vi "niScope LabVIEW Error.vi"(2 "instrument handle":u32, 3 "niScope error code (0)":i32 format="%.0x", 5 "error in (no error)":errorcluster) -> (1 "error out":errorcluster)   [LabVIEW 2013]
uses:
  niScope_32.dll
panel:
  out "VI Name":string
  out "instrument handle out":i32
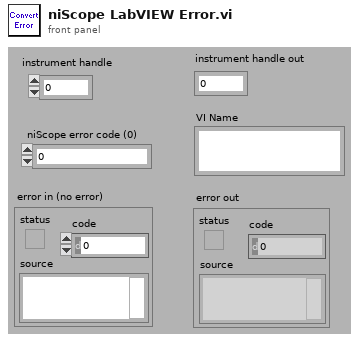
[diagram p1: front panel]
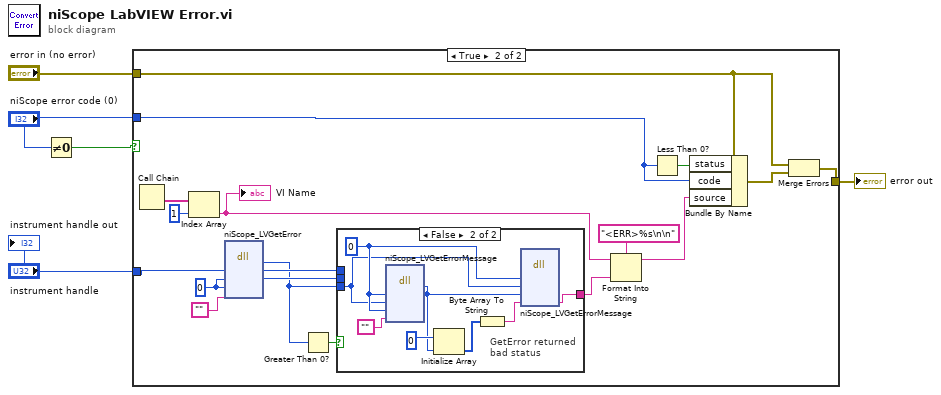
[diagram p0: block diagram]
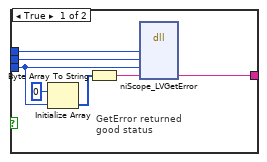
[diagram p3: hidden frame]
diagram:
  n1 = Not Equal To 0?(x="niScope error code (0)") -> (x != 0?=w1:bool)
  n2 = case shown="True" w1 {
    tunnel: "niScope error code (0)" -> [_ w15]
    tunnel: [w6 w11] -> w5
    tunnel: "instrument handle" -> [_ w14]
    tunnel: "error in (no error)" -> [w6 w13]
    frame False {
    }
    frame True {
      w21 = 0
      n3 = Call Chain() -> (call chain=w22:string[])
      n4 = Index Array(array=w22, index=1 ("Index")) -> (element=w7:string)
      "VI Name" <- w7
      n5 = dll-call lib="niScope_*.*" fn="niScope_LVGetError" label="GetError"("instrumentHandle"=w14, "errorCode"=w21, "bufferSize"=w21, "description"="") -> (w8:i32, "instrumentHandle"=w20:u32, "errorCode"=w19:i32)  [unwired: 5 in, 2 out]
      n6 = Greater Than 0?(x=w8) -> (x > 0?=w9:bool)
      n7 = case shown="False" w9 {
        tunnel: w20 -> [w28 _]
        tunnel: w19 -> [w27 _]
        tunnel: [w26 w39] -> w18
        tunnel: w8 -> [w25 w36]
        frame True {
          # "GetError returned\ngood status"
          n8 = Initialize Array(u8 0, w25) -> (w30:u8[])
          n9 = Byte Array To String(unsigned byte array=w30) -> (string=w29:string)
          n10 = dll-call lib="niScope_*.*" fn="niScope_LVGetError" label="GetError"("instrumentHandle"=w28, "errorCode"=w27, "bufferSize"=w25, "description"=w29) -> ("description"=w26:string)  [unwired: 7 in, 2 out]
        }
        frame False {
          w38 = 0 ("instrumentHandle")
          # "GetError returned\nbad status"
          n11 = dll-call lib="niScope_*.*" fn="niScope_LVGetErrorMessage" label="GetErrorMessage"("instrumentHandle"=w38, "errorCode"=w36, "bufferSize"=w38, "errorMessage"="") -> (w32:i32)  [unwired: 7 in, 2 out]
          n12 = Initialize Array(u8 0, w32) -> (w35:u8[])
          n13 = Byte Array To String(unsigned byte array=w35) -> (string=w33:string)
          n14 = dll-call lib="niScope_*.*" fn="niScope_LVGetErrorMessage" label="GetErrorMessage"("instrumentHandle"=w38, "errorCode"=w36, "bufferSize"=w32, "errorMessage"=w33) -> ("errorMessage"=w39:string)  [unwired: 7 in, 2 out]
        }
      }
      n15 = Format Into String(format string="<ERR>%s\n\n", initial string=w7, w18) -> (resulting string=w10:string)  [unwired: 1 in, 1 out]
      n16 = Less Than 0?(x=w15) -> (x < 0?=w24:bool)
      n17 = Bundle By Name(cluster=w13, "status"=w24, "code"=w15, "source"=w10) -> (w12:errorcluster)
      n18 = Merge Errors(w13, w12) -> (w11:errorcluster)
    }
  }
  "error out" <- w5
  "instrument handle out" <- "instrument handle"
